vi "Periodic Tasks.vi"(8 "error in":errorcluster) -> ()   [LabVIEW 2018]
doc: "This VI runs in parallel to other tasks. It can contain as many user-defined periodic loops as you need. These can carry out PID or other sorts of timed response."
uses:
  <vilib>/Rock Robotics/WPI/Solenoid/WPI_SolenoidValue.ctl
  <vilib>/Rock Robotics/WPI/Utilities/WPI_GetSetVariantRefNum.vi
  Robot Global Data.vi
  <vilib>/Rock Robotics/Network Tables/NT Write Number.vi
  <vilib>/Rock Robotics/Network Tables/NT Read Number.vi
  <vilib>/Rock Robotics/WPI/Solenoid/WPI_SolenoidSetEnum.vi
panel:
  out "output cluster":T1
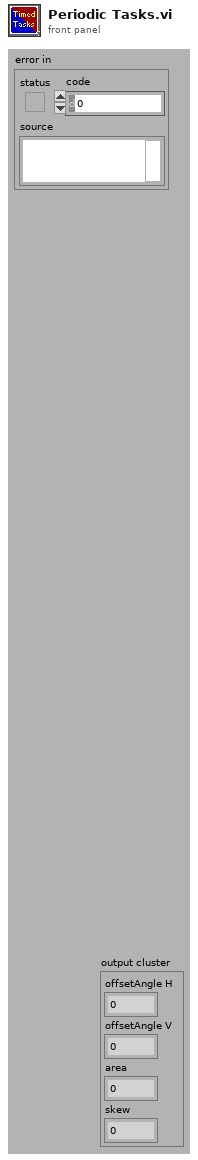
[diagram p1: front panel]
types:
  T1 = cluster{"offsetAngle H":dbl, "offsetAngle V":dbl, "area":dbl, "skew":dbl}
  T2 = typedef "WPI_RobotDriveDevRef.ctl" = cluster{"DevStatus":errorcluster, "Motors[]":T3[], "Square Inputs":bool, "Max Output":dbl}
  T3 = typedef "WPI_MotorControlDeviceRef.ctl" = cluster{"DeviceStatus":errorcluster, "Type":T4, "PWM":cluster{"PWM Channel":T5, "DeadBand":T6}, "CAN":cluster{"Device Number":u8, "SetOutput VI Ref":variant, "GetOutput VI Ref":variant, "Enable VI Ref":variant, "Disable VI Ref":variant, "Data":variant}, "Invert":bool, "DIO PWM":cluster{"PWM \"Enable\" Channel":T5, "DIOChannel":T7, "PWM Rate":dbl}}
  T4 = typedef "WPI_MotorControlType.ctl" = enum16{"PWM", "CAN", "DIO PWM"}
  T5 = typedef "FPGA_DIOPWMChannel.ctl" = enum8{"PWM 0", "PWM 1", "PWM 2", "PWM 3", "PWM 4", "PWM 5", "PWM 6", "PWM 7", "PWM 8", "PWM 9", "PWM MXP 0", "PWM MXP 1", "PWM MXP 2", "PWM MXP 3", "PWM MXP 4", "PWM MXP 5", "PWM MXP 6", "PWM MXP 7", "PWM MXP 8", "PWM MXP 9", "Invalid"}
  T6 = typedef "WPI_PWMDeadband.ctl" = cluster{"Name":string, "maxPositivePwm":i32, "minPositivePwm":i32, "centerPwm":i32, "maxNegativePwm":i32, "minNegativePwm":i32, "angularRange":u16}
  T7 = typedef "FPGA_DIOChannel.ctl" = enum8{"DIO 0", "DIO 1", "DIO 2", "DIO 3", "DIO 4", "DIO 5", "DIO 6", "DIO 7", "DIO 8", "DIO 9", "DIO MXP 0", "DIO MXP 1", "DIO MXP 2", "DIO MXP 3", "DIO MXP 4", "DIO MXP 5", "DIO MXP 6", "DIO MXP 7", "DIO MXP 8", "DIO MXP 9", "DIO MXP 10", "DIO MXP 11", "DIO MXP 12", "DIO MXP 13", "DIO MXP 14", "DIO MXP 15", "SPI Port CS1", "SPI Port CS2", "SPI Port CS3", "SPI Port MISO", "SPI Port MOSI", "Invalid"}
  T8 = typedef "WPI_JoystickDevRef.ctl" = cluster{"Device":T9}
  T9 = typedef "WPI_JoystickDeviceEnum.ctl" = enum16{"USB 0", "USB 1", "USB 2", "USB 3", "USB 4", "USB 5"}
  T10 = cluster{"JoystickDevRef":T8, "RobotDriveDevRef":T2}
  T11 = typedef "WPI_SolenoidValue.ctl" = enum16{"Off", "On", "Forward", "Reverse"}
  T12 = typedef "WPI_SolenoidDevRef.ctl" = cluster{"DevStatus":errorcluster, "Pneumatics Control Module":u8, "Forward Solenoid Channel":T13, "Reverse Solenoid Channel":T13}
  T13 = typedef "WPI_SolenoidChannel.ctl" = enum8{"Solenoid 0", "Solenoid 1", "Solenoid 2", "Solenoid 3", "Solenoid 4", "Solenoid 5", "Solenoid 6", "Solenoid 7", "Invalid"}
  T14 = typedef "WPI_GyroDevRef.ctl" = cluster{"DevStatus":errorcluster, "Analog Channel":T15, "Gain (VoltsPerDegree/Second)":dbl, "Gyro Type":enum16{"Analog", "XRS450"}, "Handle":i32, "SPI Bus":T16, "Device Found":bool, "Sample Rate":dbl, "Calibrate On Open":bool, "Offset":dbl}
  T15 = typedef "FPGA_AIChannel.ctl" = enum8{"AI 0", "AI 1", "AI 2", "AI 3", "AI MXP 0", "AI MXP 1", "AI MXP 2", "AI MXP 3", "Invalid"}
  T16 = typedef "spi_bus.ctl" = enum16{"SPI On-Board, CS0", "SPI On-Board, CS1", "SPI On-Board, CS2", "SPI On-Board, CS3", "SPI MXP", "Invalid"}
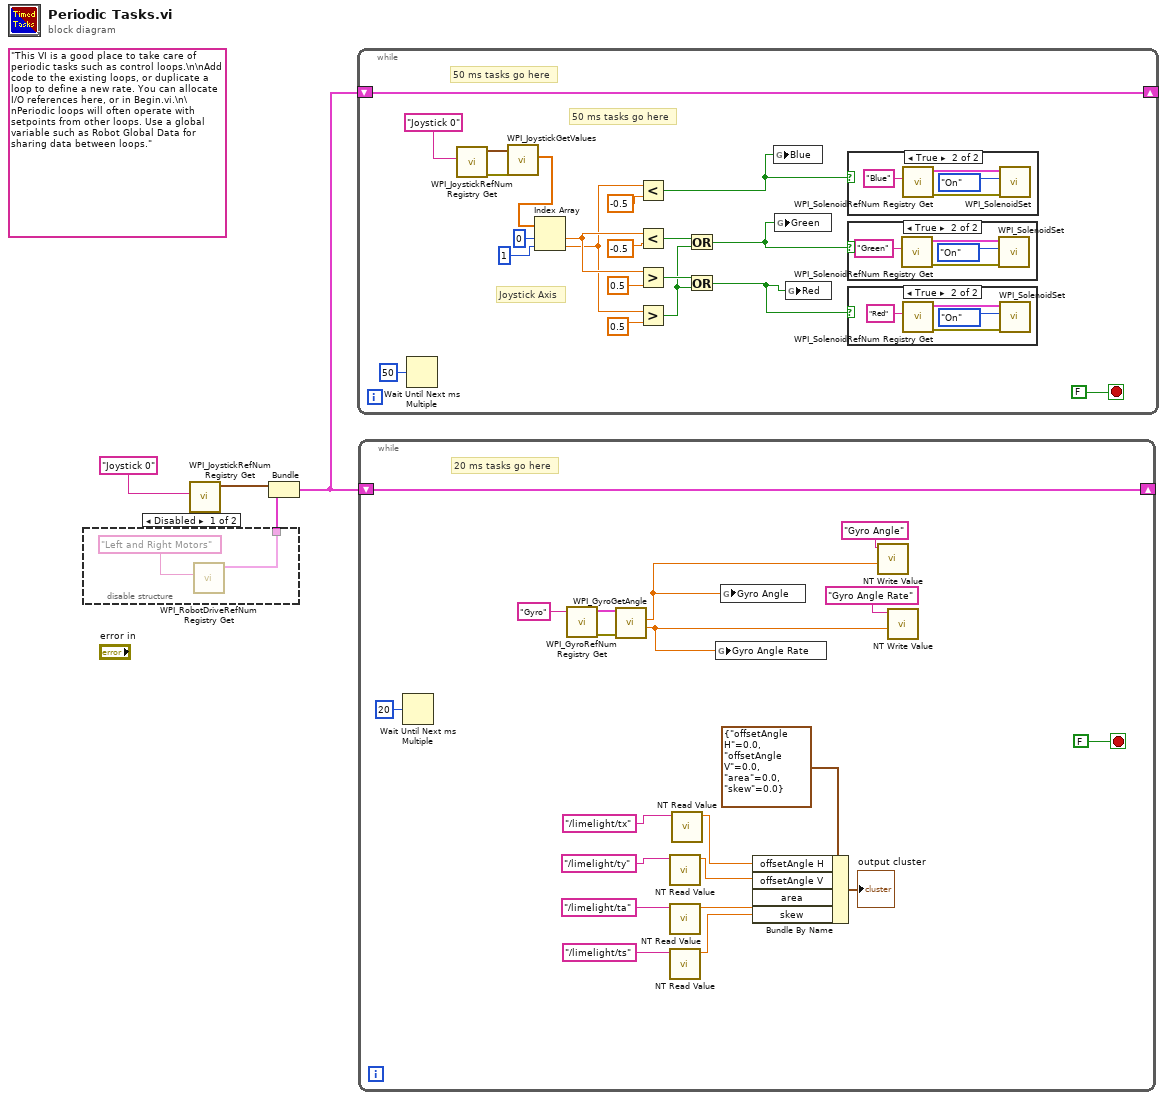
[diagram p0: block diagram]
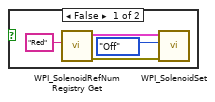
[diagram p3: hidden frame]
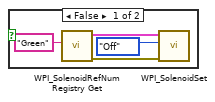
[diagram p4: hidden frame]
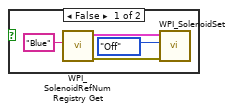
[diagram p5: hidden frame]
diagram:
  (unwired) "This VI is a good place to take care of periodic tasks such as control loops.\n\nAdd code to the existing loops, or duplicate a loop to define a new rate. You can allocate I/O references here, or in Begin.vi.\n\nPeriodic loops will often operate with setpoints from other loops. Use a global variable such as Robot Global Data for sharing data between loops."
  n1 = disable-structure shown="Disabled" {
    disable-tunnel: [w5 _] -> w2
    frame Disabled {
      n2 = call <vilib>:"WPI_RobotDriveRefNum Registry Get.vi"("refnum name"="Left and Right Motors") -> ("RobotDriveDevRef"=w5:T2)  [unwired: 1 in, 9 out]
    }
    frame Enabled {
    }
  }
  n3 = call <vilib>:"WPI_JoystickRefNum Registry Get.vi"("refnum name"="Joystick 0") -> ("JoystickDevRef"=w3:T8)  [unwired: 1 in, 9 out]
  n4 = Bundle("JoystickDevRef"=w3, "RobotDriveDevRef"=w2) -> (w1:T10)  [unwired: 1 out]
  n5 = while {
    shift-right: [w26] -> _
    shift-left: w1 -> [w26]
    stop <- FALSE stop-if-true
    # "Joystick Axis"
    # "50 ms tasks go here"
    # "50 ms tasks go here"
    n6 = Wait Until Next ms Multiple(millisecond multiple=u32 50 ("milliseconds to wait")) -> ()  [unwired: 1 out]
    n7 = call <vilib>:"WPI_JoystickRefNum Registry Get.vi"("refnum name"="Joystick 0") -> ("error out"=w11:errorcluster, "JoystickDevRef"=w12:T8)  [unwired: 1 in, 8 out]
    n8 = call <vilib>:"WPI_JoystickGetValues.vi"("error in (no error)"=w11, "JoystickDevRef"=w12) -> ("Axes"=w24:dbl[])  [unwired: 5 in, 4 out]
    n9 = Index Array(array=w24, index #1=0 ("index"), index #2=1 ("index")) -> (element #1=w14:dbl, element #2=w13:dbl)
    n10 = Less?(x=w13, y=-0.5) -> (x < y?=w9:bool)
    n11 = Less?(x=w14, y=-0.5) -> (x < y?=w20:bool)
    n12 = Greater?(x=w14, y=0.5) -> (0:w19:bool)
    n13 = Greater?(x=w13, y=0.5) -> (0:w17:bool)
    n14 = Or(x=w20, y=w17) -> (x .or. y?=w8:bool)
    n15 = Or(x=w19, y=w17) -> (x .or. y?=w7:bool)
    n16 = global write "Robot Global Data.vi" "Blue"(w9) -> ()
    n17 = global write "Robot Global Data.vi" "Green"(w8) -> ()
    n18 = global write "Robot Global Data.vi" "Red"(w7) -> ()
    n19 = case shown="True" w9 {
      frame False {
        n20 = call <vilib>:"WPI_SolenoidRefNum Registry Get.vi"("refnum name"="Blue") -> ("error out"=w47:errorcluster, "SolenoidDevRef"=w46:T12)  [unwired: 9 in]
        n21 = call-poly <vilib>:"WPI_SolenoidSet.vi"("error in (no error)"=w47, "Value"=WPI_SolenoidValue."Off", "SolenoidDevRef"=w46) -> ()  [unwired: 7 in, 2 out]
      }
      frame True {
        n22 = call <vilib>:"WPI_SolenoidRefNum Registry Get.vi"("refnum name"="Blue") -> ("error out"=w51:errorcluster, "SolenoidDevRef"=w50:T12)  [unwired: 9 in]
        n23 = call-poly <vilib>:"WPI_SolenoidSet.vi"("error in (no error)"=w51, "Value"=WPI_SolenoidValue."On", "SolenoidDevRef"=w50) -> ()  [unwired: 7 in, 2 out]
      }
    }
    n24 = case shown="True" w8 {
      frame False {
        n25 = call <vilib>:"WPI_SolenoidRefNum Registry Get.vi"("refnum name"="Green") -> ("error out"=w39:errorcluster, "SolenoidDevRef"=w38:T12)  [unwired: 9 in]
        n26 = call-poly <vilib>:"WPI_SolenoidSet.vi"("error in (no error)"=w39, "Value"=WPI_SolenoidValue."Off", "SolenoidDevRef"=w38) -> ()  [unwired: 7 in, 2 out]
      }
      frame True {
        n27 = call <vilib>:"WPI_SolenoidRefNum Registry Get.vi"("refnum name"="Green") -> ("error out"=w43:errorcluster, "SolenoidDevRef"=w42:T12)  [unwired: 9 in]
        n28 = call-poly <vilib>:"WPI_SolenoidSet.vi"("error in (no error)"=w43, "Value"=WPI_SolenoidValue."On", "SolenoidDevRef"=w42) -> ()  [unwired: 7 in, 2 out]
      }
    }
    n29 = case shown="True" w7 {
      frame False {
        n30 = call <vilib>:"WPI_SolenoidRefNum Registry Get.vi"("refnum name"="Red") -> ("error out"=w31:errorcluster, "SolenoidDevRef"=w30:T12)  [unwired: 9 in]
        n31 = call-poly <vilib>:"WPI_SolenoidSet.vi"("error in (no error)"=w31, "Value"=WPI_SolenoidValue."Off", "SolenoidDevRef"=w30) -> ()  [unwired: 7 in, 2 out]
      }
      frame True {
        n32 = call <vilib>:"WPI_SolenoidRefNum Registry Get.vi"("refnum name"="Red") -> ("error out"=w35:errorcluster, "SolenoidDevRef"=w34:T12)  [unwired: 9 in]
        n33 = call-poly <vilib>:"WPI_SolenoidSet.vi"("error in (no error)"=w35, "Value"=WPI_SolenoidValue."On", "SolenoidDevRef"=w34) -> ()  [unwired: 7 in, 2 out]
      }
    }
  }
  n34 = while {
    shift-right: [w70] -> _
    shift-left: w1 -> [w70]
    stop <- FALSE stop-if-true
    # "20 ms tasks go here"
    n35 = Wait Until Next ms Multiple(millisecond multiple=u32 20 ("milliseconds to wait")) -> ()  [unwired: 1 out]
    n36 = call <vilib>:"WPI_GyroRefNum Registry Get.vi"("refnum name"="Gyro") -> ("error out"=w67:errorcluster, "GyroDevRef"=w66:T14)  [unwired: 9 in]
    n37 = call <vilib>:"WPI_GyroGetAngle.vi"("error in"=w67, "GyroDevRef"=w66) -> ("Angular Rate"=w62:dbl, "Angle"=w63:dbl)  [unwired: 5 in, 3 out]
    n38 = call-poly <vilib>:"NT Read Value.vi"("Name"="/limelight/ty" ("refnum name")) -> ("Numeric"=w56:dbl)  [unwired: 9 in, 1 out]
    n39 = call-poly <vilib>:"NT Read Value.vi"("Name"="/limelight/ta" ("refnum name")) -> ("Numeric"=w55:dbl)  [unwired: 9 in, 1 out]
    n40 = call-poly <vilib>:"NT Read Value.vi"("Name"="/limelight/ts" ("refnum name")) -> ("Numeric"=w54:dbl)  [unwired: 9 in, 1 out]
    n41 = call-poly <vilib>:"NT Read Value.vi"("Name"="/limelight/tx" ("refnum name")) -> ("Numeric"=w57:dbl)  [unwired: 9 in, 1 out]
    n42 = global write "Robot Global Data.vi" "Gyro Angle Rate"(w62) -> ()
    n43 = global write "Robot Global Data.vi" "Gyro Angle"(w63) -> ()
    n44 = Bundle By Name(cluster=T1 {"offsetAngle H"=0.0, "offsetAngle V"=0.0, "area"=0.0, "skew"=0.0} ("input cluster"), "offsetAngle H"=w57, "offsetAngle V"=w56, "area"=w55, "skew"=w54) -> (→"output cluster":T1)
    n45 = call-poly <vilib>:"NT Write Value.vi"("Numeric"=w63, "Name"="Gyro Angle") -> ()  [unwired: 9 in, 1 out]
    n46 = call-poly <vilib>:"NT Write Value.vi"("Numeric"=w62, "Name"="Gyro Angle Rate") -> ()  [unwired: 9 in, 1 out]
  }
